vi "PH_Sequencer.check for MA MM1.vi"(1 "Heads":T1[](array[typedef])) -> (0 "MA MM1 must be set?":bool)   [LabVIEW 2014, in "PH_Sequencer.lvlib"]
uses:
  PH_Sequencer.lvlib
  PH_BeamlineInformation/PH_BeamlineInformation.Head.ctl
  PH_Basics/PH_PP_Common/PH_PP_Common.PUs.ctl
  PH_BeamlineInformation/PH_BeamlineInformation.lvlib
  PH_Basics/PH_PP_Common/PH_PP_Common.lvlib
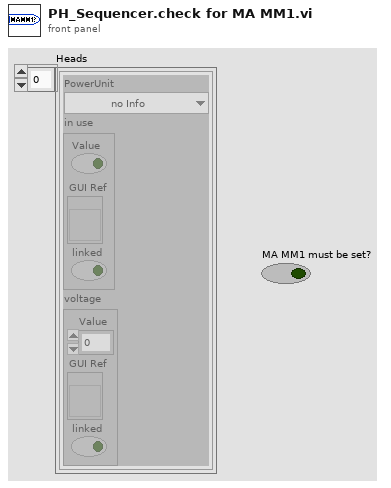
[diagram p1: front panel]
types:
  T1 = typedef "PH_BeamlineInformation.lvlib/PH_BeamlineInformation.Head.ctl" = cluster{"PowerUnit":T2, "in use":cluster{"Value":bool, "GUI Ref":refnum<vi>, "linked":bool}, "voltage":cluster{"Value":dbl, "GUI Ref":refnum<vi>, "linked":bool}}
  T2 = typedef "PH_PP_Common.lvlib/PH_PP_Common.PUs.ctl" = enum16{"no Info", "PA-19mm-1", "PA-19mm-2", "PA-45mm-PILC", "PA-45mm-MAIN", "MA-PU-1", "MA-PU-2", "MA-PU-3", "MA-PU-4", "MA-PU-5", "MA-PU-6", "MA-FR", "MA-PILC", "PA-45mm-DP"}
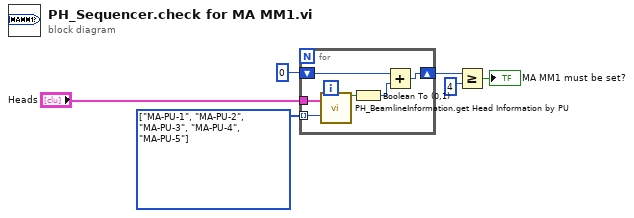
[diagram p0: block diagram]
diagram:
  w5 = T2[] [enum."MA-PU-1", enum."MA-PU-2", enum."MA-PU-3", enum."MA-PU-4", enum."MA-PU-5"] items=["no Info", "PA-19mm-1", "PA-19mm-2", "PA-45mm-PILC", "PA-45mm-MAIN", "MA-PU-1", "MA-PU-2", "MA-PU-3", "MA-PU-4", "MA-PU-5", "MA-PU-6", "MA-FR", "MA-PILC", "PA-45mm-DP"]
  n1 = for {
    tunnel: "Heads" -> [w12]
    tunnel: w5 -> [w11] mode=indexing
    shift-right: [w8] -> w1
    shift-left: i16 0 -> [w7]
    n2 = call "PH_BeamlineInformation.get Head Information by PU.vi"("Heads"=w12, "Power Unit"=w11) -> ("In Use?"=w10:bool)  [unwired: 12 in, 5 out]
    n3 = Boolean To (0,1)(Boolean=w10) -> (0, 1=w9:i16)
    n4 = Add(x=w7, y=w9) -> (x+y=w8:i16)
  }
  n5 = Greater Or Equal?(x=w1, y=i16 4) -> (x >= y?=→"MA MM1 must be set?":bool)
